vi "close visa.vi"(8 "error in (no error)":errorcluster, 11 "Simulado in":refnum<class "Simulado.lvclass">) -> (0 "error out":errorcluster, 3 "Simulado out":refnum<class "Simulado.lvclass">)   [LabVIEW 2020, in "Simulado.lvclass"]
uses:
  Simulado.lvclass
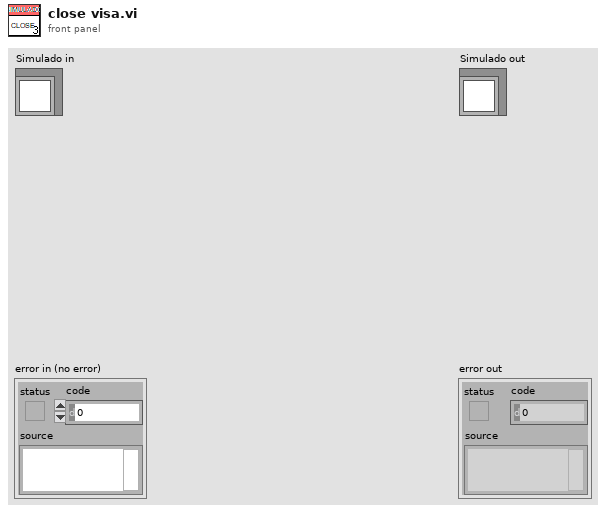
[diagram p1: front panel]
types:
  T1 = enum16{"reset parameters", "Get parameters", "Set parameter"}
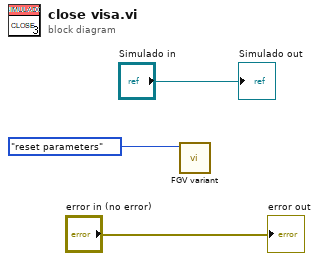
[diagram p0: block diagram]
diagram:
  n1 = call "FGV variant.vi"("Functions"=T1."reset parameters") -> ()  [unwired: 9 in, 2 out]
  "error out" <- "error in (no error)"
  "Simulado out" <- "Simulado in"
